vi "Config Voltage After Close Outlet.vi"(8 "error in (no error)":errorcluster, 10 "Voltage":dbl, 11 "FPGA API Concrete in":refnum<class "FPGA API Concrete.lvclass">) -> (0 "error out":errorcluster, 3 "FPGA API Concrete out":refnum<class "FPGA API Concrete.lvclass">)   [LabVIEW 2019, in "FPGA API Concrete.lvclass"]
uses:
  FPGA API Concrete.lvclass
  FPGA API Concrete.lvclass/FPGA API Concrete.ctl
  <vilib>/Utility/error.llb/Error Cluster From Error Code.vi
  <vilib>/rvi/errors/niLvFpgaAdjustHostInterfaceError.vi
  <vilib>/rvi/interface/nirviReadWriteControl/nirviReadWriteControl.xnode
  FPGA Ref.ctl
  NiFpgaLv.dll
  <vilib>/rvi/interface/Simulation/niFpgaSimulationCallBeginRW.vi
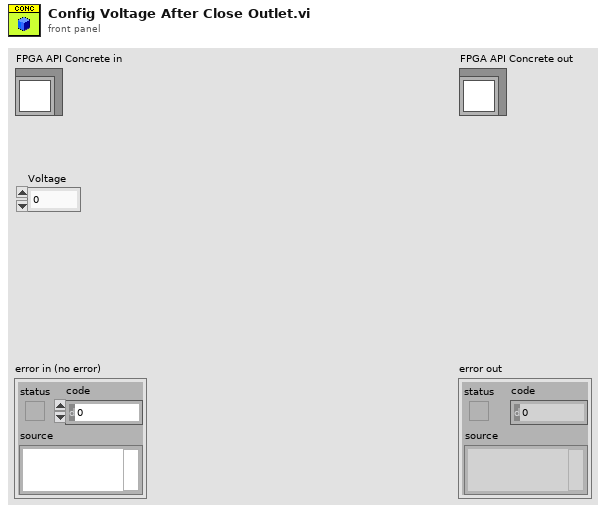
[diagram p1: front panel]
types:
  T1 = typedef "FPGA API Concrete.lvclass/FPGA Ref.ctl" = refnum<k20>
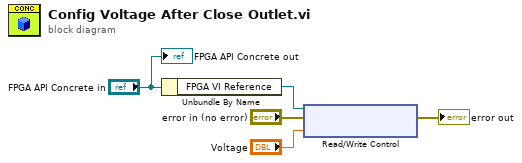
[diagram p0: block diagram]
diagram:
  n1 = Unbundle By Name("FPGA API Concrete in") -> ("FPGA VI Reference"=w4:T1)
  n2 = xnode "Read/Write Control"("FPGA VI Reference In"=w4, "error in"="error in (no error)", "VoltageAfterClose"="Voltage") -> ("error out"=→"error out":errorcluster)  [unwired: 1 out]
  "FPGA API Concrete out" <- "FPGA API Concrete in"
